vi "Event Handler.vi"(0 "uService Template in":refnum<class "Dummy.lvclass">, 5 "Event type":T1=enum."Message", 7 "Item Name":string, 9 "Data":variant, 11 "error in (no error)":errorcluster) -> (4 "uService Template out":refnum<class "Dummy.lvclass">, 15 "error out":errorcluster)   [LabVIEW 2020, in "Dummy.lvlib" / "Dummy.lvclass"]
doc: "This VI is the event handler of the uService: every time an event is triggered to the uService, this VI is called.\nNote: here you can access the Actor/Class data, but it will be the one coming out from Init. You cannot modify the values.\nThree different events are supported:\nI) Button Pressed: get called on a GUI button pressed. Item Name is the name (label) of the button, Data is empty.\nII) Shared Variable Updated: get called when a SV you subscribed to is updated. Item Name is the name of the SV, and Data is the value (note: you need to convert it to the proper type).\nIII) Message: get called every time a user event is generated using Send Message to Event Handler. The values of Item Name and Data are the one given to the Send Message to Event Handler.\nIV) Ready to launch?: this frame get called every time a new Run is initiated. Each uService is responsible of performing a self check before giving back the green light for the Run to start."
uses:
  Dummy.lvclass
  C:/LabVIEW Code/aegis-labview-code/TALOS/TALOS_PPL.lvlibp/Ancestor/Ancestor/Ancestor.lvclass
  TALOS/TALOS_PPL.lvlibp/Father of all uServices/Father of all uServices/Event Handler Items.ctl
  TALOS/TALOS_PPL.lvlibp/Ancestor/Ancestor/Read ID.vi
  TALOS/TALOS_PPL.lvlibp/Father of all uServices/Father of all uServices/Father of all uServices.lvclass
  C:/LabVIEW Code/aegis-labview-code/TALOS/TALOS_PPL.lvlibp/Father of all uServices/Father of all uServices/Father of all uServices.lvclass
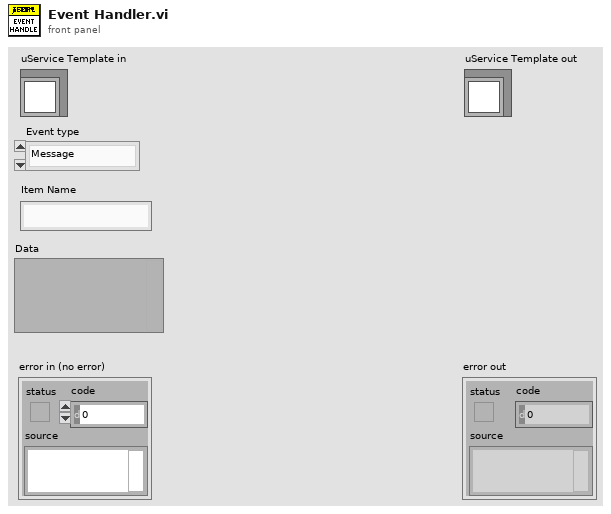
[diagram p1: front panel]
types:
  T1 = typedef "TALOS_PPL.lvlibp/Father of all uServices.lvlib/Father of all uServices.lvclass/Event Handler Items.ctl" = enum16{"Button Pressed", "Shared Variable Updated", "Message", "Ready to launch?", "Safe Mode", "Start RUN", "Stop RUN"}
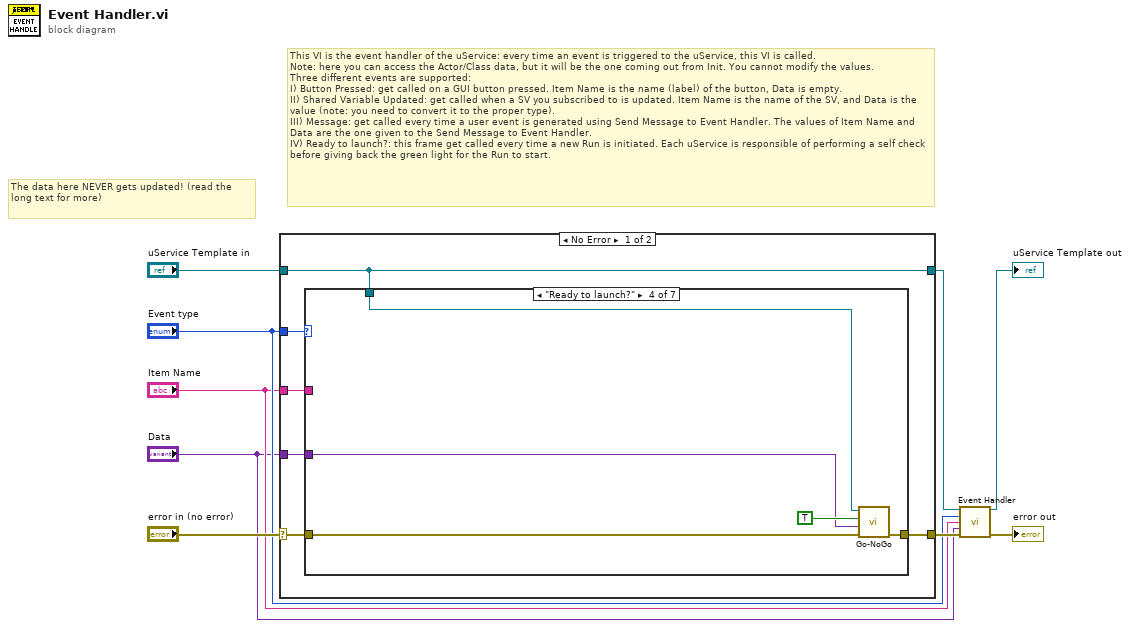
[diagram p0: block diagram]
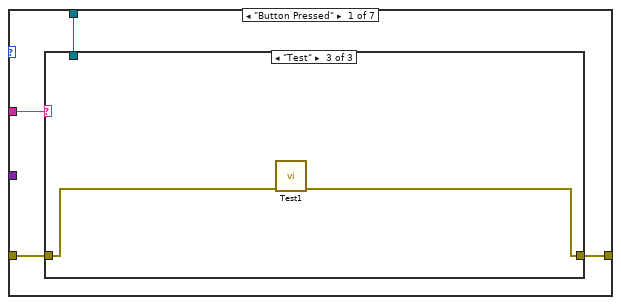
[diagram p2: hidden frame]
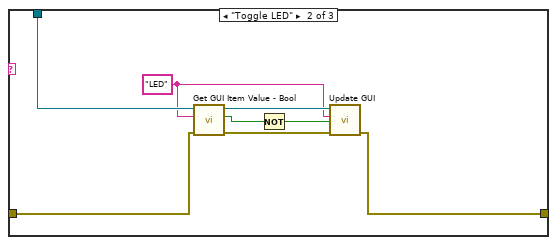
[diagram p4: hidden frame]
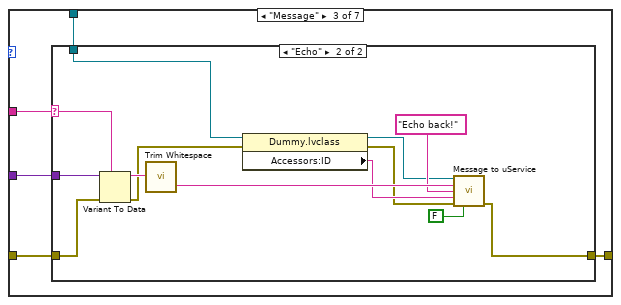
[diagram p6: hidden frame]
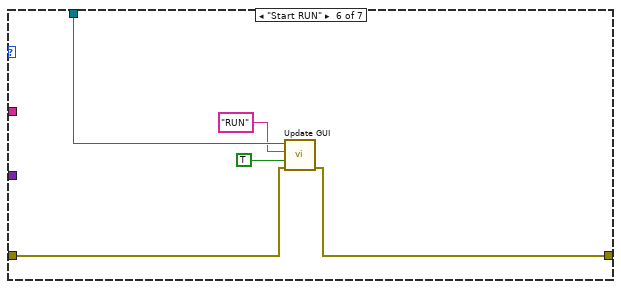
[diagram p9: hidden frame]
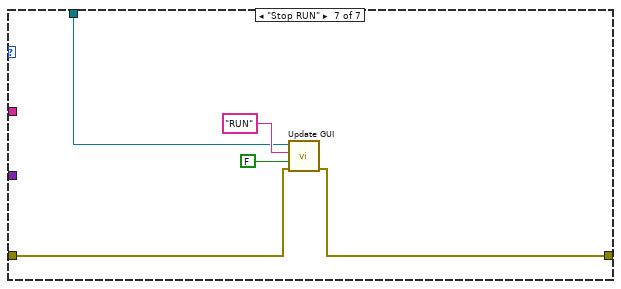
[diagram p10: hidden frame]
diagram:
  # "The data here NEVER gets updated! (read the long text for more)"
  # "This VI is the event handler of the uService: every time an event is triggered to the uService, this VI is called.\nNote: here you can access the Actor/Class data, but it will be the one coming out from Init. You cannot modify the values.\nThree different events are supported:\nI) Button Pressed: get called on a GUI button pressed. Item Name is the name (label) of the button, Data is empty.\nII) Shared Variable Updated: get called when a SV you subscribed to is updated. Item Name is the name of the SV, and Data is the value (note: you need to convert it to the proper type).\nIII) Message: get called every time a user event is generated using Send Message to Event Handler. The values of Item Name and Data are the one given to the Send Message to Event Handler.\nIV) Ready to launch?: this frame get called every time a new Run is initiated. Each uService is responsible of performing a self check before giving back the green light for the Run to start."
  n1 = case shown="No Error" "error in (no error)" {
    selector: "error in (no error)" -> [w13 w68]
    tunnel: [w14 w68] -> w7
    tunnel: [w12 w67] -> w4
    tunnel: "uService Template in" -> [w12 w67]
    tunnel: "Event type" -> [w15 _]
    tunnel: "Item Name" -> [w11 _]
    tunnel: "Data" -> [w10 _]
    frame No Error {
      n2 = case shown="\"Ready to launch?\"" w15 {
        tunnel: [w19 w31 w32 w54 w56 w58 w63] -> w14
        tunnel: w13 -> [w16 w31 w36 w55 w56 w57 w62]
        tunnel: w11 -> [w17 _ w35 _ _ _ _]
        tunnel: w12 -> [w18 _ w33 w53 _ w61 w64]
        tunnel: w10 -> [_ _ w34 w51 _ _ _]
        frame "Button Pressed" {
          n3 = case shown="\"Test\"" w17 {
            tunnel: w16 -> [w20 w21 w30]
            tunnel: [w20 w22 w29] -> w19
            tunnel: w18 -> [_ w26 _]
            frame Default {
            }
            frame "Toggle LED" {
              w25 = "LED" ("FP Item Name")
              n4 = call "Get GUI Item Value - Bool.vi"("error in (no error)"=w21, "FP Item Name"=w25, "uService Template in"=w26) -> ("error out"=w28:errorcluster, "Value"=w24:bool, "uService Template out"=w27:refnum<class "Dummy.lvclass">)  [unwired: 6 in]
              n5 = Not(x=w24) -> (.not. x?=w23:bool)
              n6 = call "Update GUI.vi"("error in (no error)"=w28, "Data"=w23, "GUI Item Name"=w25, "uService Template in"=w27) -> ("error out"=w22:errorcluster)  [unwired: 6 in, 1 out]
            }
            frame "Test" {
              n7 = call "Test1.vi"("error in (no error)"=w30) -> ("error out"=w29:errorcluster)  [unwired: 10 in]
            }
          }
        }
        frame "Shared Variable Updated" {
        }
        frame "Message" {
          n8 = case shown="\"Echo\"" w35 {
            selector: w35 -> [_ w49]
            tunnel: w36 -> [w37 w41]
            tunnel: w34 -> [_ w50]
            tunnel: w33 -> [_ w42]
            tunnel: [w37 w45] -> w32
            frame Default {
            }
            frame "Echo" {
              n9 = Variant To Data(error in=w41, type=w49, Variant=w50) -> (data=w48:string, error out=w40:errorcluster)
              n10 = call <vilib>:"Trim Whitespace.vi"("string"=w48) -> ("trimmed string"=w47:string)  [unwired: 1 in]
              n11 = property class="Dummy.lvclass"(reference=w42, error in=w40) -> (reference out=w43:refnum<class "Dummy.lvclass">, error out=w38:errorcluster, "Accessors:ID"=w39:string)
              n12 = call "Message to uService.vi"("Father of all uServices in"=w43, "uService ID"=w47, "Message"="Echo back!", "Data"=w39, "error in (no error)"=w38, "Locale?"=FALSE) -> ("error out"=w45:errorcluster)  [unwired: 8 in, 1 out]
            }
          }
        }
        frame "Ready to launch?" {
          n13 = call-dynamic "Go-NoGo.vi"("error in (no error)"=w55, "Go-NoGo Data"=w51, "Go?"=TRUE, "Father of all uServices in"=w53) -> ("error out"=w54:errorcluster)  [unwired: 6 in, 1 out]
        }
        frame "Safe Mode" {
        }
        frame "Start RUN" {
          n14 = call "Update GUI.vi"("error in (no error)"=w57, "Data"=TRUE, "GUI Item Name"="RUN", "uService Template in"=w61) -> ("error out"=w58:errorcluster)  [unwired: 6 in, 1 out]
        }
        frame "Stop RUN" {
          n15 = call "Update GUI.vi"("error in (no error)"=w62, "Data"=FALSE, "GUI Item Name"="RUN", "uService Template in"=w64) -> ("error out"=w63:errorcluster)  [unwired: 6 in, 1 out]
        }
      }
    }
    frame Error {
    }
  }
  n16 = call-parent "Event Handler.vi"("uService Template in"=w4, "Event type"="Event type", "Item Name"="Item Name", "Data"="Data", "error in (no error)"=w7) -> ("uService Template out"=→"uService Template out":refnum<class "Dummy.lvclass">, "error out"=→"error out":errorcluster)  [unwired: 9 in]
